vi "Construct.vi"(8 "error in (no error)":errorcluster, 11 "ErrorManager in":refnum<class "ErrorManager.lvclass">) -> (0 "error out":errorcluster, 3 "ErrorManager out":refnum<class "ErrorManager.lvclass">)   [LabVIEW 2020, in "ErrorManager.lvlib" / "ErrorManager.lvclass"]
uses:
  ErrorManager.lvclass
  ErrorInfo.ctl
  obj/Addons/LabVIEWObjectInterfaces.lvlibp/ErrorManager/ErrorManager/ErrorType.ctl
  ErrorManager.lvclass/ErrorManager.ctl
  obj/Addons/LabVIEWObjectInterfaces.lvlibp/LabVIEWObjectInterfaces/IErrorManager/IErrorManager.lvclass
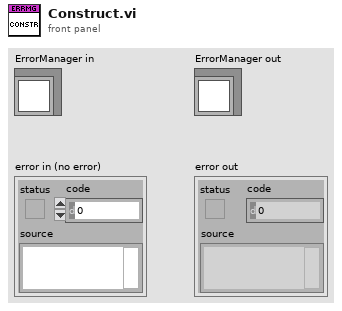
[diagram p1: front panel]
types:
  T1 = typedef "ErrorManager.lvlib/ErrorManager.lvclass/ErrorInfo.ctl" = cluster{"Time Stamp":timestamp, "Message":string, "Type":T2}
  T2 = typedef "LabVIEWObjectInterfaces.lvlibp/IErrorManager.lvclass/ErrorType.ctl" = enum16{"Info", "Warning", "Error"}
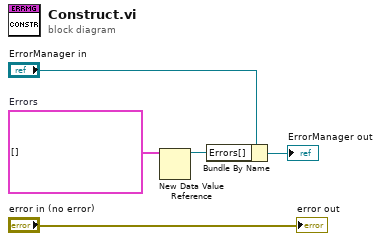
[diagram p0: block diagram]
diagram:
  w4 = T1[] []  # Errors
  n1 = New Data Value Reference(data value=w4) -> (data value reference=w3:refnum<data-value>)  [unwired: 1 in, 1 out]
  n2 = Bundle By Name(cluster="ErrorManager in", "Errors[]"=w3) -> (→"ErrorManager out":refnum<class "ErrorManager.lvclass">)
  "error out" <- "error in (no error)"
